vi "drift_pixel2m (SubVI).vi"(0 "Application in":refnum<vi>, 1 "X drift":i32, 2 "Y drift":i32, 3 "error in":errorcluster, 5 "Drift correction Pixels":i32) -> (6 "Application out":refnum<vi>, 7 "x drift":sgl, 8 "y drift":sgl, 9 "error out":errorcluster)   [LabVIEW 2014]
uses:
  <userlib>/Nanonis Prog Interface V5/Nanonis Prog Interface.lvlib
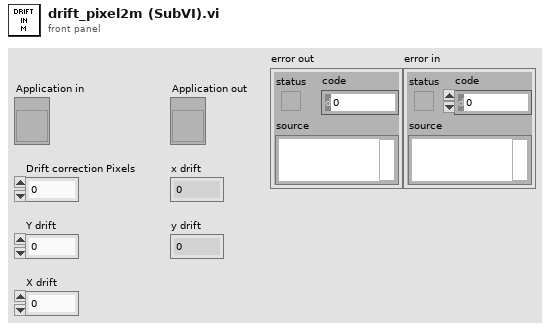
[diagram p1: front panel]
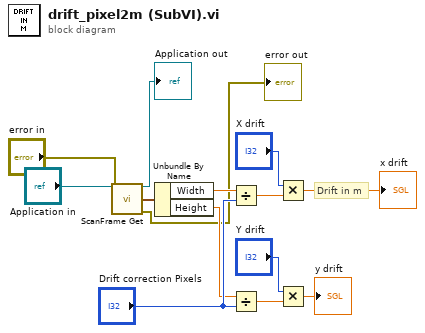
[diagram p0: block diagram]
diagram:
  # "Drift in m"
  n1 = call <userlib>:"ScanFrame Get.vi"("Application ref in"="Application in", "error in (no error)"="error in") -> ("Application ref out"=→"Application out":refnum<vi>, "Size (m)"=w4:cluster{"Width":sgl, "Height":sgl}, "error out"=→"error out":errorcluster)  [unwired: 9 in, 2 out]
  n2 = Unbundle By Name(w4) -> ("Width"=w5:sgl, "Height"=w3:sgl)
  n3 = Divide(x=w5, y="Drift correction Pixels") -> (x/y=w6:sgl)
  n4 = Divide(x=w3, y="Drift correction Pixels") -> (x/y=w7:sgl)
  n5 = Multiply(x="X drift", y=w6) -> (x*y=→"x drift":sgl)
  n6 = Multiply(x="Y drift", y=w7) -> (x*y=→"y drift":sgl)
